vi "Vision Processing.vi"(4 "error in (no error)":errorcluster, 6 "CameraDevRef":T1) -> ()   [LabVIEW 2011]
uses:
  <vilib>/Rock Robotics/WPI/Camera/WPI_CameraDevRef.ctl
  Robot Global Data.vi
  <vilib>/vision/NI_Vision_Development_Module.lvlib
panel:
  in  "Max Distance for 1 hoop":dbl=8.0
  out "Raw Turret":dbl
  in  "Run Calculations":bool
  out "Target X Coord":dbl
  out "Target Distance":dbl
  out "Target Y Coord":dbl
  out "Distance Array":dbl[](array[numeric])
  in  "Scaler":dbl=0.85
  in  "Lower Speed Limit":dbl=0.05
  out "Number of Rectangles Visible":dbl
  out "Y Position Array":dbl[](array[numeric])
  out "X Position Array":dbl[](array[numeric])
  in  "View":bool
  out "Target Info":T2(array[cluster])
  in  "Area Size Limit":i32=444
  in  "Particle Count Limit":i32=8
  in  "Score Limits":T3={"Rect Coverage"=76.0, "Aspect Ratio"=40.0, "X Edge Strength"=40.0, "Y Edge Strength"=60.0}
  in  "Processing":enum32{"Color", "Intensity", "Intensity Open"}(tab)=enum."Intensity"
  in  "Luminance":i32=255
  in  "Saturation":i32=255
  in  "Hue":i32(knob)=65 scale=0.0..255.0
  in  "Margins":cluster{"Hue":i32, "Sat":i32, "Lum":i32}={"Hue"=20, "Sat"=27, "Lum"=30} {"Sat" scale=0.0..40.0; "Lum" scale=0.0..40.0; "Hue" scale=0.0..40.0}
  in  "Range":cluster{"Lower value":sgl, "Upper value":sgl}={"Lower value"=107.17391, "Upper value"=255.0} {"Lower value" scale=0.0..255.0; "Upper value" scale=0.0..255.0}
  in  "Range":cluster{"Lower value":sgl, "Upper value":sgl}={"Lower value"=123.804344, "Upper value"=255.0} {"Lower value" scale=0.0..255.0; "Upper value" scale=0.0..255.0}
  in  "View":bool
  out "Processed Image":T4(plugin-control)
  out "Original Image":T4(plugin-control)
  # "Instructions:\nProcessing the reflective tape that is illuminated by a ring light can be based\non color or light intensity.\nParticles within the image are scored by rectangle coverage, aspect ratio, and\nfor being hollow with a bold edge. A particle is considered a target if all scores\nare above the score limits. Particles can be annotated -- surrounded by\na rectangle and scores drawn to the left .\nTo control the number of particles being scored, use the count limit and the size\nlimit."
  # "(in)"
  # "To debug, Enable using the View button.\nFor color processing, you can click in the image to select the color for processing."
  # "Enable by clicking the View button.\nGreen scores are above the limit, orange are below. Inner/outer rect\nindicates all passed."
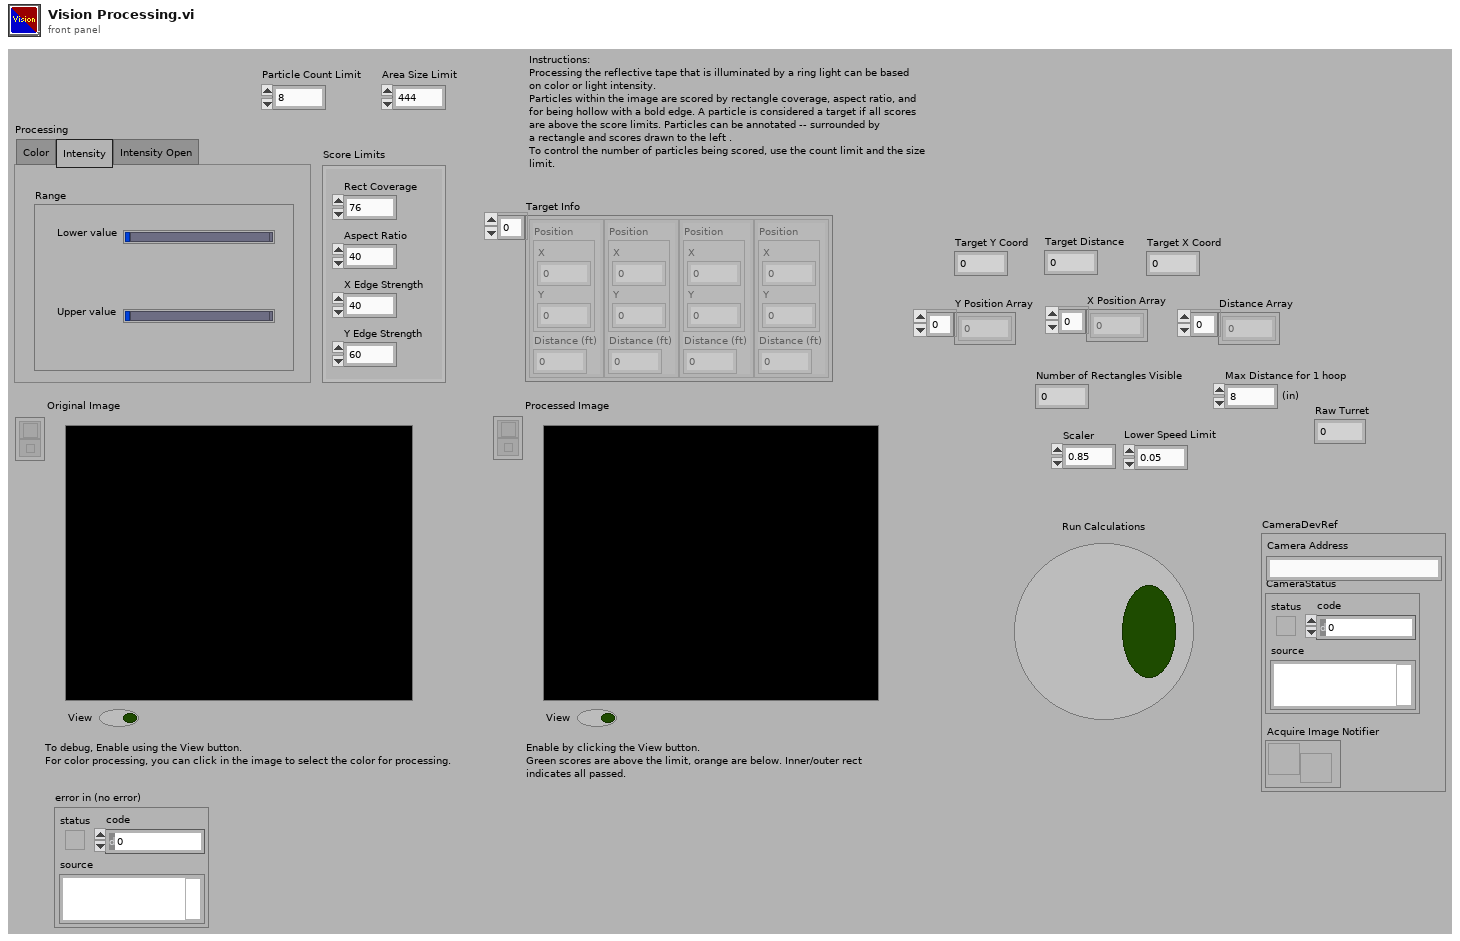
[diagram p1: front panel]
types:
  T1 = typedef "WPI_CameraDevRef.ctl" = cluster{"Camera Address":string, "CameraStatus":errorcluster, "Acquire Image Notifier":refnum<notifier>}
  T2 = cluster{"Position":cluster{"X":dbl, "Y":dbl}, "Distance (ft)":dbl}[]
  T3 = cluster{"Rect Coverage":dbl, "Aspect Ratio":dbl, "X Edge Strength":dbl, "Y Edge Strength":dbl}
  T4 = typedef "IMAQ Image.ctl" = refnum<image>
  T5 = typedef "Image Type" = u32
  T6 = enum32{"AutoM", "Close", "Dilate", "Erode", "Gradient", "Gradient out", "Gradient in", "Hit miss", "Open", "PClose", "POpen", "Thick", "Thin"}
  T7 = typedef "WPI_CameraImageSize.ctl" = enum16{"640x480", "320x240", "160x120"}
  T8 = cluster{"fps":i32, "compression":i32, "Image Size":T7}
  T9 = cluster{cluster{"Left":dbl, "Top":dbl, "Right":dbl, "Bottom":dbl}, dbl[]}[]
  T10 = cluster{"Left":dbl, "Top":dbl, "Right":dbl, "Bottom":dbl}
  T11 = cluster{"Target Center (-1 to 1)":cluster{"X":dbl, "Y":dbl}, "Distance (ft)":dbl}
  T12 = cluster{"Target Center (-1 to 1)":cluster{"X":dbl, "Y":dbl}, "Distance (ft)":dbl}[]
  T13 = typedef "WPI_JoystickDevRef.ctl" = cluster{"Device":T14}
  T14 = typedef "WPI_JoystickDeviceEnum.ctl" = enum16{"USB 1", "USB 2", "USB 3", "USB 4", "Kinect 1", "Kinect 2"}
  T15 = typedef "WPI_JoystickButtonState.ctl" = cluster{"Button 1":bool, "Button 2":bool, "Button 3":bool, "Button 4":bool, "Button 5":bool, "Button 6":bool, "Button 7":bool, "Button 8":bool, "Button 9":bool, "Button 10":bool, "Button 11":bool, "Button 12":bool}
  T16 = cluster{"axis 1 (x)":dbl, "axis 2 (y)":dbl, "axis 3 (throttle)":dbl, "axis 4":dbl, "axis 5":dbl, "axis 6":dbl}
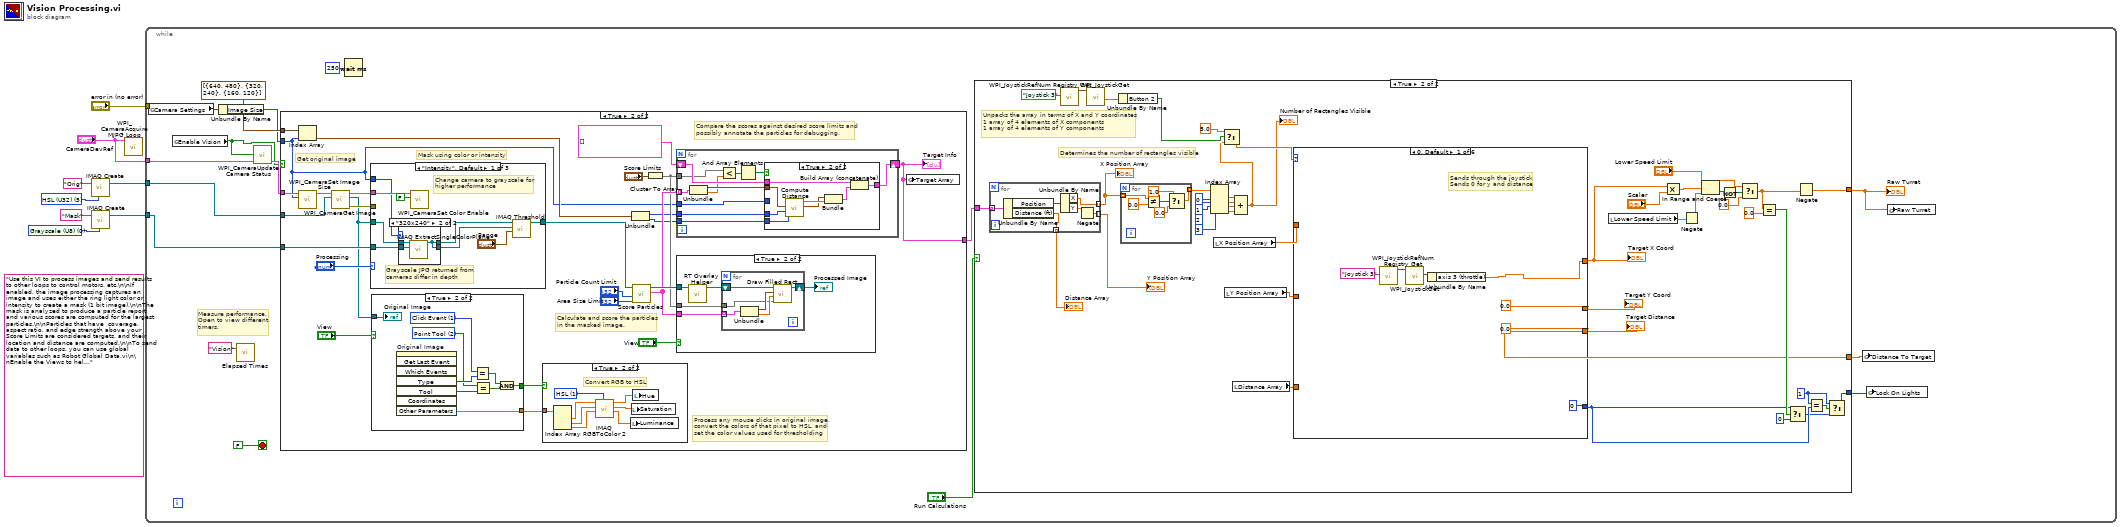
[diagram p0: block diagram]
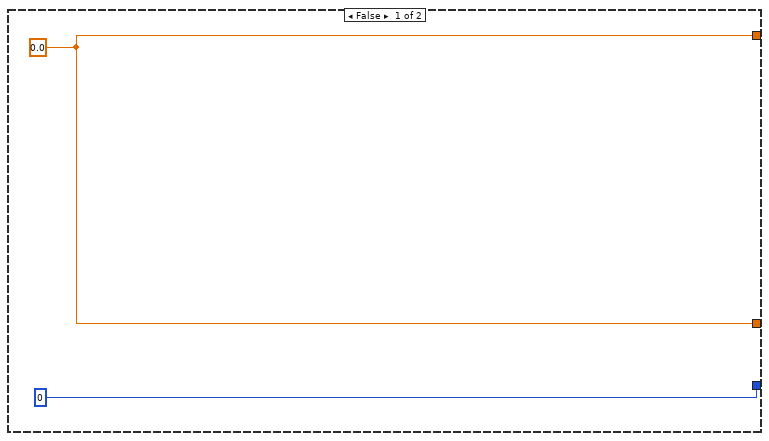
[diagram p2: hidden frame]
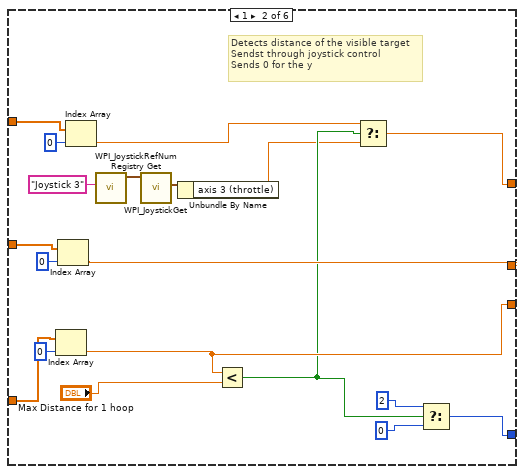
[diagram p3: hidden frame]
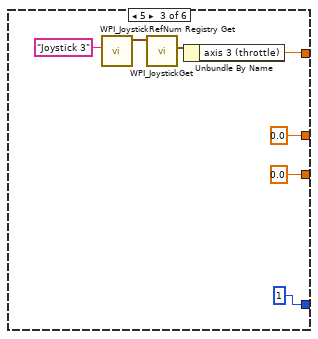
[diagram p4: hidden frame]
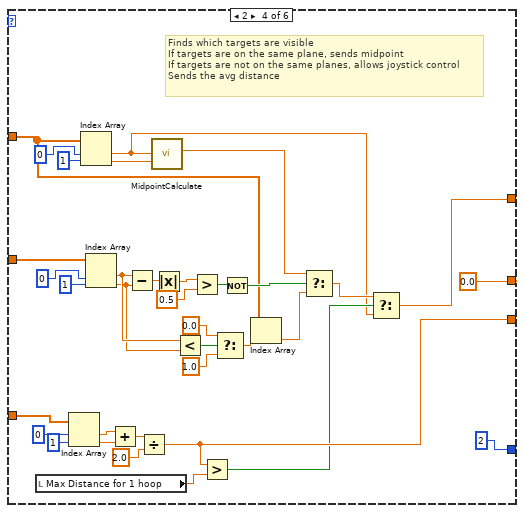
[diagram p5: hidden frame]
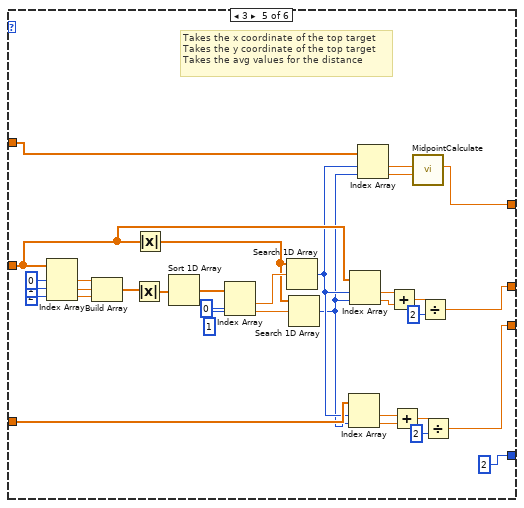
[diagram p6: hidden frame]
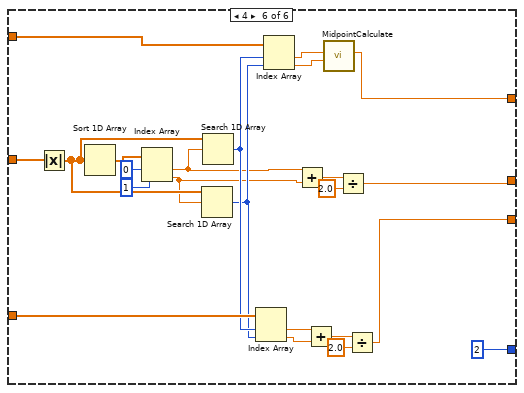
[diagram p7: hidden frame]
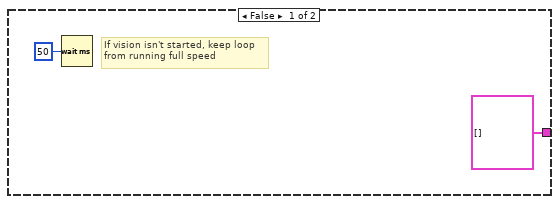
[diagram p8: hidden frame]
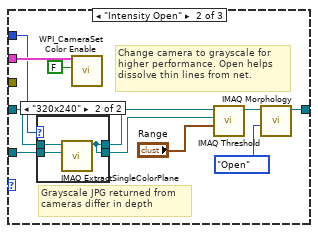
[diagram p11: hidden frame]
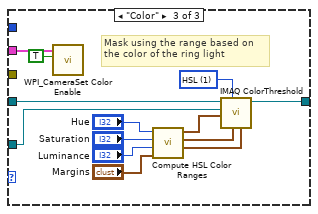
[diagram p13: hidden frame]
diagram:
  w3 = T5 0 items=["Grayscale (U8)", "Grayscale (I16)", "Grayscale (SGL)", "Complex (CSG)", "RGB (U32)", "HSL (U32)", "RGB (U64)", "Grayscale (U16)"] ("Image Type")
  (unwired) "Use this VI to process images and send results to other loops to control motors, etc.\n\nIf enabled, the image processing captures an image and uses either the ring light color or intensity to create a mask (1 bit image).\n\nThe mask is analyzed to produce a particle report and various scores are computed for the largest particles.\n\nParticles that have  coverage, aspect ratio, and edge strength above your Score Limits are considered targets, and their location and distance are computed.\n\nTo send data to other loops, you can use global variables such as Robot Global Data.vi\n\nEnable the Views to help debug color settings. Disable the View to speed up processing."
  w7 = T5 5 items=["Grayscale (U8)", "Grayscale (I16)", "Grayscale (SGL)", "Complex (CSG)", "RGB (U32)", "HSL (U32)", "RGB (U64)", "Grayscale (U16)"] ("Image Type")
  n1 = call "IMAQ Create"("Image Name"="Orig", "Image Type"=w7) -> ("New Image"=w6:T4)  [unwired: 2 in, 2 out]
  n2 = call "IMAQ Create"("Image Name"="Mask", "Image Type"=w3) -> ("New Image"=w1:T4)  [unwired: 2 in, 2 out]
  n3 = call <vilib>:"WPI_CameraAcquire MJPG Loop.vi"("CameraDevRef"="CameraDevRef") -> ()  [unwired: 11 in]
  n4 = while {
    tunnel: w6 -> [w23]
    tunnel: "CameraDevRef" -> [w22]
    tunnel: "error in (no error)" -> [_]
    tunnel: w1 -> [w18]
    stop <- FALSE stop-if-true
    # "Measure performance.\nOpen to view different\ntimers."
    n5 = global read "Robot Global Data.vi" "Camera Settings"() -> (w16:T8)
    n6 = global read "Robot Global Data.vi" "Enable Vision"() -> (w20:bool)
    n7 = Unbundle By Name(w16) -> ("Image Size"=w15:T7)
    n8 = call "Elapsed Times.vi"("Call Name"="Vision") -> ()  [unwired: 2 in, 1 out]
    n9 = call <vilib>:"WPI_CameraUpdate Camera Status.vi"("CameraDevRef In"=w22, "Enable Vision"=w20) -> ("CameraDevRef Out"=w21:T1)  [unwired: 3 in]
    n10 = case shown="True" w20 {
      tunnel: w23 -> [_ w225]
      tunnel: w21 -> [_ w221]
      tunnel: w18 -> [_ w212]
      tunnel: cluster{i32, i32}[] [{640, 480}, {320, 240}, {160, 120}] -> [_ w216]
      tunnel: w15 -> [_ w209]
      tunnel: [T2 [] w210] -> w14
      frame False {
        # "If vision isn't started, keep loop\nfrom running full speed"
        n11 = Wait (ms)(milliseconds to wait=u32 50) -> ()  [unwired: 1 out]
      }
      frame True {
        # "Compare the scores against desired score limits and\npossibly annotate the particles for debugging."
        # "Process any mouse clicks in original image,\nconvert the colors of that pixel to HSL, and\nset the color values used for thresholding"
        # "Calculate and score the particles\nin the masked image."
        # "Mask using color or intensity"
        # "Get original image"
        n12 = call <vilib>:"WPI_CameraSet Image Size.vi"("Image Size"=w209, "CameraDevRef"=w221) -> ("CameraDevRef Out"=w222:T1)  [unwired: 8 in, 1 out]
        n13 = Index Array(array=w216, index=w209) -> (element=w213:cluster{i32, i32})
        n14 = call <vilib>:"WPI_CameraGet Image.vi"("Image"=w225, "CameraDevRef"=w222) -> ("error out"=w223:errorcluster, "Image Out"=w211:T4, "CameraDevRef Out"=w224:T1)  [unwired: 7 in]
        n15 = case shown="\"Intensity\", Default" "Processing" {
          tunnel: w211 -> [w247 w259 w285]
          tunnel: [w250 w264 w284] -> w219
          tunnel: w224 -> [w248 w262 w275]
          tunnel: w223 -> [_ _ _]
          tunnel: w212 -> [w246 w260 w273]
          tunnel: w209 -> [w245 w261 _]
          frame "Intensity", Default {
            # "Grayscale JPG returned from\ncameras differ in depth"
            # "Change camera to grayscale for\nhigher performance"
            n16 = case shown="\"320x240\"" w245 {
              tunnel: w247 -> [w253 w256]
              tunnel: w246 -> [w252 w255]
              tunnel: [w253 w254] -> w244
              tunnel: [w252 w254] -> w243
              frame "640x480", Default {
              }
              frame "320x240" {
                n17 = call "IMAQ ExtractSingleColorPlane"("Image Dst"=w255, "Image Src"=w256) -> ("Image Dst Out"=w254:T4)  [unwired: 8 in, 1 out]
              }
            }
            n18 = call <vilib>:"WPI_CameraSet Color Enable.vi"("Color Enabled"=FALSE, "CameraDevRef"=w248) -> ()  [unwired: 8 in, 2 out]
            n19 = call "IMAQ Threshold"("Range"="Range", "Image Dst"=w243, "Image Src"=w244) -> ("Image Dst Out"=w250:T4)  [unwired: 3 in, 5 out]
          }
          frame "Intensity Open" {
            # "Grayscale JPG returned from\ncameras differ in depth"
            # "Change camera to grayscale for\nhigher performance. Open helps\ndissolve thin lines from net."
            n20 = case shown="\"320x240\"" w261 {
              tunnel: w259 -> [w269 w272]
              tunnel: w260 -> [w268 w271]
              tunnel: [w269 w270] -> w258
              tunnel: [w268 w270] -> w257
              frame "640x480", Default {
              }
              frame "320x240" {
                n21 = call "IMAQ ExtractSingleColorPlane"("Image Dst"=w271, "Image Src"=w272) -> ("Image Dst Out"=w270:T4)  [unwired: 8 in, 1 out]
              }
            }
            n22 = call <vilib>:"WPI_CameraSet Color Enable.vi"("Color Enabled"=FALSE, "CameraDevRef"=w262) -> ()  [unwired: 8 in, 2 out]
            n23 = call "IMAQ Threshold"("Range"="Range", "Image Dst"=w257, "Image Src"=w258) -> ("Image Dst Out"=w265:T4)  [unwired: 3 in, 5 out]
            n24 = call "IMAQ Morphology"("Operation"=T6."Open", "Image Src"=w265) -> ("Image Dst Out"=w264:T4)  [unwired: 8 in, 1 out]
          }
          frame "Color" {
            w283 = u16 1 items=["RGB", "HSL", "HSV", "HSI"] ("Color Mode")
            # "Mask using the range based on\nthe color of the ring light"
            n25 = call <vilib>:"WPI_CameraSet Color Enable.vi"("Color Enabled"=TRUE, "CameraDevRef"=w275) -> ()  [unwired: 8 in, 2 out]
            n26 = call "Compute HSL Color Ranges.vi"("Margins"="Margins", "Luminance"="Luminance", "Saturation"="Saturation", "Hue"="Hue") -> ("Lum Range"=w280:cluster{i32, i32}, "Sat Range"=w281:cluster{i32, i32}, "Hue Range"=w282:cluster{i32, i32})  [unwired: 5 in]
            n27 = call "IMAQ ColorThreshold"("Blue or Luma or Val or Inten Range"=w280, "Green or Sat Range"=w281, "Color Mode"=w283, "Red or Hue Range"=w282, "Image Dst"=w273, "Image Src"=w285) -> ("Image Dst Out"=w284:T4)  [unwired: 4 in, 1 out]
          }
        }
        n28 = case shown="True" "View" {
          tunnel: w211 -> [_ w305]
          tunnel: [_ w300] -> w218
          tunnel: [_ w297] -> w217
          frame False {
          }
          frame True {
            w298 = 2 items=["None", "Selection Tool", "Point Tool", "Line Tool", "Rectangle Tool", "Oval Tool", "Polygon Tool", "ClosedFreehandTool", "Annulus Tool", "Rotated Rectangle Tool", "Zoom Tool", "Pan Tool", "Polyline Tool", "Freehand Tool"] ("Tool")
            w299 = 1 items=["No Event"=0, "Click Event"=1, "Draw Event"=2, "Size Event"=4, "Scroll Event"=5, "Double Click Event"=8] ("Type")
            n29 = invoke on="Original Image" class="ImageControl" method="Get Last Event"() -> ("Type"=w301:i32, "Tool"=w304:i32, "Other Parameters"=w297:sgl[])  [unwired: 8 in, 5 out]
            n30 = Equal?(x=w299, y=w301) -> (x = y?=w302:bool)
            n31 = Equal?(x=w298, y=w304) -> (x = y?=w303:bool)
            n32 = And(x=w302, y=w303) -> (x .and. y?=w300:bool)
            "Original Image" <- w305
          }
        }
        n33 = case shown="True" w218 {
          tunnel: w217 -> [_ w242]
          frame False {
          }
          frame True {
            w241 = u16 1 items=["RGB", "HSL", "HSV", "HSI", "CIE L*a*b*", "CIE XYZ"] ("Color Mode")
            # "Convert RGB to HSL"
            n34 = Index Array(array=w242) -> (element #1=w240:sgl, element #2=w238:sgl, element #3=w236:sgl)  [unwired: 3 in]
            n35 = call "IMAQ RGBToColor 2"("Color Mode"=w241, "Blue value"=w236, "Green value"=w238, "Red value"=w240) -> ("Blue or Luma or Val or Inten or Z or b*value"=w235:dbl, "Green or Sat or Y or a* value"=w237:dbl, "Red or Hue or X or L* value"=w239:dbl)  [unwired: 4 in, 1 out]
            n36 = local write "Luminance"(w235) -> ()
            n37 = local write "Saturation"(w237) -> ()
            n38 = local write "Hue"(w239) -> ()
          }
        }
        n39 = Unbundle(w213) -> (w215:i32, w214:i32)
        n40 = call "Score Particles.vi"("Area Size Limit"="Area Size Limit", "Particle Count Limit"="Particle Count Limit", "Image Refnum in"=w219) -> ("Scored Particle Info"=w230:T9, "Image Refnum out"=w233:T4)  [unwired: 7 in]
        n41 = Cluster To Array(cluster="Score Limits") -> (array=w228:dbl[])
        n42 = for {
          shift-right: [w315] -> w210
          shift-left: T2 [] -> [w316]
          tunnel: w215 -> [w314]
          tunnel: w230 -> [w312] mode=indexing
          tunnel: w228 -> [w307]
          tunnel: w209 -> [w311]
          tunnel: w214 -> [w306]
          n43 = Unbundle(w312) -> (w313:T10, w308:dbl[])
          n44 = Less?(x=w307, y=w308) -> (x < y?=w310:bool[])
          n45 = And Array Elements(Boolean array=w310) -> (logical AND=w309:bool)
          n46 = case shown="True" w309 {
            tunnel: w316 -> [w317 w325]
            tunnel: [w317 w324] -> w315
            tunnel: w313 -> [_ w320]
            tunnel: w314 -> [_ w322]
            tunnel: w311 -> [_ _]
            tunnel: w306 -> [_ w319]
            frame False {
            }
            frame True {
              n47 = call "Compute Distance.vi"("Y Image Resolution"=w319, "X Image Resolution"=w322, "Bounding Box"=w320) -> ("Target Center (-1 to 1)"=w318:cluster{"X":dbl, "Y":dbl}, "Distance (ft)"=w321:dbl)  [unwired: 7 in]
              n48 = Bundle("Target Center (-1 to 1)"=w318, "Distance (ft)"=w321) -> (w323:T11)  [unwired: 1 in]
              n49 = Build Array (concatenate)(w325, w323) -> (w324:T12)
            }
          }
        }
        "Target Info" <- w210
        n50 = case shown="True" "View" {
          tunnel: w233 -> [_ w287]
          tunnel: w230 -> [_ w289]
          tunnel: w228 -> [_ w288]
          frame False {
          }
          frame True {
            n51 = call "RT Overlay Helper.vi"("Refnum in"=w287) -> ("Refnum out"=w290:T4)  [unwired: 10 in]
            n52 = for {
              shift-right: [w295] -> w286
              shift-left: w290 -> [w296]
              tunnel: w289 -> [w292] mode=indexing
              tunnel: w288 -> [w291]
              n53 = Unbundle(w292) -> (w293:T10, w294:dbl[])
              n54 = call "Draw Filled Rect.vi"("Limits"=w291, "Scores"=w294, "Bounding Box"=w293, "image in"=w296) -> ("image out"=w295:T4)  [unwired: 7 in]
            }
            "Processed Image" <- w286
          }
        }
        n55 = global write "Robot Global Data.vi" "Target Array"(w210) -> ()
      }
    }
    n56 = Wait (ms)(milliseconds to wait=u32 250) -> ()  [unwired: 1 out]
    n57 = case shown="True" "Run Calculations" {
      tunnel: w14 -> [_ w43]
      tunnel: [w25 w27] -> w11
      tunnel: [0 ("f") w35] -> w10
      tunnel: [w25 w30] -> w9
      frame False {
        w25 = 0.0 ("f")
      }
      frame True {
        w36 = 1 ("y")
        # "Determines the number of rectangles visible"
        # "Unpacks the array in terms of X and Y coordinates\n1 array of 4 elements of X components\n1 array of 4 elements of Y components"
        n58 = for {
          tunnel: [w204] -> w44 mode=indexing
          tunnel: [w205] -> w54 mode=indexing
          tunnel: w43 -> [w202] mode=indexing
          tunnel: [w201] -> w63 mode=indexing
          n59 = Unbundle By Name(w202) -> ("Position"=w206:cluster{"X":dbl, "Y":dbl}, "Distance (ft)"=w201:dbl)
          n60 = Unbundle By Name(w206) -> ("X"=w205:dbl, "Y"=w203:dbl)
          n61 = Negate(x=w203) -> (-x=w204:dbl)
        }
        "X Position Array" <- w54
        "Y Position Array" <- w44
        "Distance Array" <- w63
        n62 = call <vilib>:"WPI_JoystickRefNum Registry Get.vi"("refnum name"="Joystick 3") -> ("JoystickDevRef"=w41:T13)  [unwired: 9 in, 1 out]
        n63 = call <vilib>:"WPI_JoystickGet.vi"("JoystickDevRef"=w41) -> ("Buttons"=w39:T15)  [unwired: 4 in, 2 out]
        n64 = Unbundle By Name(w39) -> ("Button 2"=w38:bool)
        n65 = for {
          tunnel: w54 -> [w75] mode=indexing
          tunnel: [w71] -> w53 mode=indexing
          n66 = Not Equal?(x=w75, y=0.0) -> (x != y?=w74:bool)
          n67 = Select(t=1.0, s=w74, f=0.0) -> (s? t:f=w71:dbl)
        }
        n68 = Index Array(array=w53, index #1=0 ("index"), index #2=1 ("index"), index #3=2 ("index"), index #4=3 ("index")) -> (element #1=w51:dbl, element #2=w52:dbl, element #3=w50:dbl, element #4=w49:dbl)
        n69 = local read "X Position Array"() -> (w55:dbl[])
        n70 = local read "Y Position Array"() -> (w66:dbl[])
        n71 = local read "Distance Array"() -> (w67:dbl[])
        n72 = Compound Arithmetic op=ADD(w51, w52, w50, w49) -> (w29:dbl)
        "Number of Rectangles Visible" <- w29
        n73 = Select(t=5.0, s=w38, f=w29) -> (s? t:f=w69:dbl)
        n74 = case shown="0, Default" w69 {
          tunnel: w55 -> [_ w99 _ w118 w161 w195]
          tunnel: [w77 w92 w103 w111 w158 w185] -> w65
          tunnel: [0.0 ("X") w89 0.0 ("X") 0.0 ("X") w162 w184] -> w64
          tunnel: [0.0 ("X") w95 0.0 ("X") w115 w146 w179] -> w30
          tunnel: w66 -> [_ w90 _ w142 w154 w200]
          tunnel: w67 -> [_ w102 _ w128 w149 w194]
          tunnel: [0 w85 1 2 2 2] -> w33
          frame 0, Default {
            # "Sends through the joystick\nSends 0 for y and distance"
            n75 = call <vilib>:"WPI_JoystickRefNum Registry Get.vi"("refnum name"="Joystick 3") -> ("JoystickDevRef"=w81:T13)  [unwired: 9 in, 1 out]
            n76 = call <vilib>:"WPI_JoystickGet.vi"("JoystickDevRef"=w81) -> ("Axes"=w79:T16)  [unwired: 4 in, 2 out]
            n77 = Unbundle By Name(w79) -> ("axis 3 (throttle)"=w77:dbl)
          }
          frame 1 {
            # "Detects distance of the visible target\nSendst through joystick control\nSends 0 for the y"
            n78 = Index Array(array=w102, index=0) -> (element=w95:dbl)
            n79 = Index Array(array=w90, index=0) -> (element=w89:dbl)
            n80 = Index Array(array=w99, index=0) -> (element=w93:dbl)
            n81 = call <vilib>:"WPI_JoystickRefNum Registry Get.vi"("refnum name"="Joystick 3") -> ("JoystickDevRef"=w98:T13)  [unwired: 9 in, 1 out]
            n82 = call <vilib>:"WPI_JoystickGet.vi"("JoystickDevRef"=w98) -> ("Axes"=w96:T16)  [unwired: 4 in, 2 out]
            n83 = Unbundle By Name(w96) -> ("axis 3 (throttle)"=w84:dbl)
            n84 = Less?(x=w95, y="Max Distance for 1 hoop") -> (x < y?=w87:bool)
            n85 = Select(t=w93, s=w87, f=w84) -> (s? t:f=w92:dbl)
            n86 = Select(t=2, s=w87, f=0) -> (s? t:f=w85:i32)
          }
          frame 5 {
            n87 = call <vilib>:"WPI_JoystickRefNum Registry Get.vi"("refnum name"="Joystick 3") -> ("JoystickDevRef"=w107:T13)  [unwired: 9 in, 1 out]
            n88 = call <vilib>:"WPI_JoystickGet.vi"("JoystickDevRef"=w107) -> ("Axes"=w105:T16)  [unwired: 4 in, 2 out]
            n89 = Unbundle By Name(w105) -> ("axis 3 (throttle)"=w103:dbl)
          }
          frame 2 {
            # "Finds which targets are visible\nIf targets are on the same plane, sends midpoint\nIf targets are not on the same planes, allows joystick control\nSends the avg distance"
            n90 = local read "Max Distance for 1 hoop"() -> (w114:dbl)
            n91 = Index Array(array=w128, index #1=0 ("index"), index #2=1 ("index")) -> (element #1=w127:dbl, element #2=w126:dbl)
            n92 = Index Array(array=w118, index #1=0 ("index"), index #2=1 ("index")) -> (element #1=w110:dbl, element #2=w132:dbl)
            n93 = Index Array(array=w142, index #1=0 ("index"), index #2=1 ("index")) -> (element #1=w124:dbl, element #2=w123:dbl)
            n94 = Add(x=w127, y=w126) -> (x+y=w131:dbl)
            n95 = Subtract(x=w124, y=w123) -> (x-y=w139:dbl)
            n96 = Divide(x=w131, y=2.0) -> (x/y=w115:dbl)
            n97 = call "MidpointCalculate.vi"("X2"=w132, "X1"=w110) -> ("Midpoint"=w134:dbl)  [unwired: 9 in]
            n98 = Absolute Value(x=w139) -> (abs(x)=w138:dbl)
            n99 = Less?(x=w124, y=w123) -> (x < y?=w122:bool)
            n100 = Greater?(x=w138, y=0.5) -> (0:w135:bool)
            n101 = Greater?(x=w115, y=w114) -> (0:w113:bool)
            n102 = Select(t=0.0, s=w122, f=1.0) -> (s? t:f=w119:dbl)
            n103 = Not(x=w135) -> (.not. x?=w136:bool)
            n104 = Index Array(array=w118, index=w119) -> (element=w117:dbl)
            n105 = Select(t=w134, s=w136, f=w117) -> (s? t:f=w112:dbl)
            n106 = Select(t=w112, s=w113, f=w110) -> (s? t:f=w111:dbl)
          }
          frame 3 {
            # "Takes the x coordinate of the top target\nTakes the y coordinate of the top target\nTakes the avg values for the distance"
            n107 = Index Array(array=w154, index #1=0 ("index"), index #2=1 ("index"), index #3=2 ("index")) -> (element #1=w174:dbl, element #2=w173:dbl, element #3=w172:dbl)
            n108 = Build Array(w174, w173, w172) -> (w171:dbl[])
            n109 = Absolute Value(x=w171) -> (abs(x)=w165:dbl[])
            n110 = Absolute Value(x=w154) -> (abs(x)=w157:dbl[])
            n111 = Sort 1D Array(array=w165) -> (sorted array=w170:dbl[])
            n112 = Index Array(array=w170, index #1=0 ("index"), index #2=1 ("index")) -> (element #1=w166:dbl, element #2=w167:dbl)
            n113 = Search 1D Array(1D array=w157, element=w166) -> (index of element=w148:i32)  [unwired: 1 in]
            n114 = Search 1D Array(1D array=w157, element=w167) -> (index of element=w147:i32)  [unwired: 1 in]
            n115 = Index Array(array=w149, index #1=w148, index #2=w147) -> (element #1=w151:dbl, element #2=w150:dbl)
            n116 = Index Array(array=w154, index #1=w148, index #2=w147) -> (element #1=w156:dbl, element #2=w155:dbl)
            n117 = Index Array(array=w161, index #1=w148, index #2=w147) -> (element #1=w160:dbl, element #2=w159:dbl)
            n118 = Add(x=w156, y=w155) -> (x+y=w164:dbl)
            n119 = Add(x=w151, y=w150) -> (x+y=w152:dbl)
            n120 = call "MidpointCalculate.vi"("X2"=w159, "X1"=w160) -> ("Midpoint"=w158:dbl)  [unwired: 9 in]
            n121 = Divide(x=w164, y=2) -> (x/y=w162:dbl)
            n122 = Divide(x=w152, y=2) -> (x/y=w146:dbl)
          }
          frame 4 {
            n123 = Absolute Value(x=w200) -> (abs(x)=w196:dbl[])
            n124 = Sort 1D Array(array=w196) -> (sorted array=w199:dbl[])
            n125 = Index Array(array=w199, index #1=0 ("index"), index #2=1 ("index")) -> (element #1=w191:dbl, element #2=w190:dbl)
            n126 = Search 1D Array(1D array=w196, element=w190) -> (index of element=w192:i32)  [unwired: 1 in]
            n127 = Search 1D Array(1D array=w196, element=w191) -> (index of element=w193:i32)  [unwired: 1 in]
            n128 = Index Array(array=w194, index #1=w193, index #2=w192) -> (element #1=w181:dbl, element #2=w180:dbl)
            n129 = Index Array(array=w195, index #1=w193, index #2=w192) -> (element #1=w187:dbl, element #2=w186:dbl)
            n130 = Add(x=w191, y=w190) -> (x+y=w189:dbl)
            n131 = Add(x=w181, y=w180) -> (x+y=w182:dbl)
            n132 = call "MidpointCalculate.vi"("X2"=w186, "X1"=w187) -> ("Midpoint"=w185:dbl)  [unwired: 9 in]
            n133 = Divide(x=w189, y=2.0) -> (x/y=w184:dbl)
            n134 = Divide(x=w182, y=2.0) -> (x/y=w179:dbl)
          }
        }
        "Target Y Coord" <- w64
        "Target Distance" <- w30
        "Target X Coord" <- w65
        n135 = local read "Lower Speed Limit"() -> (w57:dbl)
        n136 = Multiply(x=w65, y="Scaler") -> (x*y=w62:dbl)
        n137 = Negate(x=w57) -> (-x=w58:dbl)
        n138 = In Range and Coerce(upper limit="Lower Speed Limit", x=w62, lower limit=w58) -> (In Range?=w59:bool)  [unwired: 1 out]
        n139 = Not(x=w59) -> (.not. x?=w60:bool)
        n140 = Select(t=w62, s=w60, f=0.0) -> (s? t:f=w28:dbl)
        n141 = Equal?(x=w28, y=0.0) -> (x = y?=w34:bool)
        n142 = Select(t=w33, s=w34, f=0) -> (s? t:f=w31:i32)
        n143 = Negate(x=w28) -> (-x=w27:dbl)
        n144 = Equal?(x=w36, y=w33) -> (x = y?=w37:bool)
        n145 = Select(t=w36, s=w37, f=w31) -> (s? t:f=w35:i32)
      }
    }
    "Raw Turret" <- w11
    n146 = global write "Robot Global Data.vi" "Distance To Target"(w9) -> ()
    n147 = global write "Robot Global Data.vi" "Lock On Lights"(w10) -> ()
    n148 = global write "Robot Global Data.vi" "Raw Turret"(w11) -> ()
  }
